vi "Read Max.vi"(8 "error in (no error)":errorcluster, 11 "Stats_I64_CIF_U in":refnum<class "Stats_I64_CIF_U.lvclass">) -> (0 "error out":errorcluster, 2 "Max":i64, 3 "Stats_I64_CIF_U out":refnum<class "Stats_I64_CIF_U.lvclass">)   [LabVIEW 2021, in "Stats_CIF_U.lvlib" / "Stats_I64_CIF_U.lvclass"]
uses:
  Stats_I64_CIF_U.lvclass
  Stats_I64_CIF_U.lvclass/Stats_I64_CIF_U.ctl
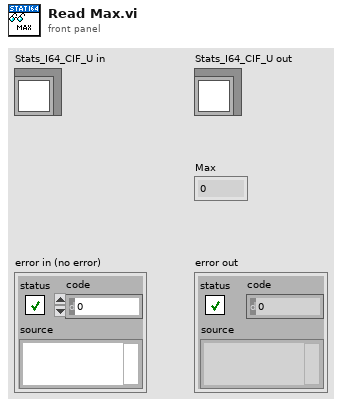
[diagram p1: front panel]
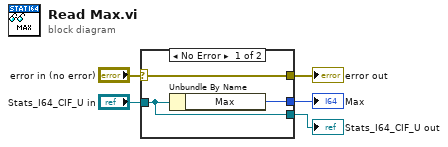
[diagram p0: block diagram]
diagram:
  n1 = case shown="No Error" "error in (no error)" {
    selector: "error in (no error)" -> [w8 w9]
    tunnel: [w8 w9] -> w4
    tunnel: [w7 w10] -> w2
    tunnel: "Stats_I64_CIF_U in" -> [w7 w10]
    tunnel: [w6 _] -> w1
    frame No Error {
      n2 = Unbundle By Name(w7) -> ("Max"=w6:i64)
    }
    frame Error {
    }
  }
  "error out" <- w4
  "Stats_I64_CIF_U out" <- w2
  "Max" <- w1
